vi "Read Points.vi"(8 "error in (no error)":errorcluster, 11 "Locus Recorder in":refnum<class "Locus Recorder.lvclass">) -> (0 "error out":errorcluster, 2 "Points":dbl[][](array[numeric]), 3 "Locus Recorder out":refnum<class "Locus Recorder.lvclass">)   [LabVIEW 2014, in "Locus Recorder.lvclass"]
uses:
  Locus Recorder.lvclass
  Locus Recorder.lvclass/Locus Recorder.ctl
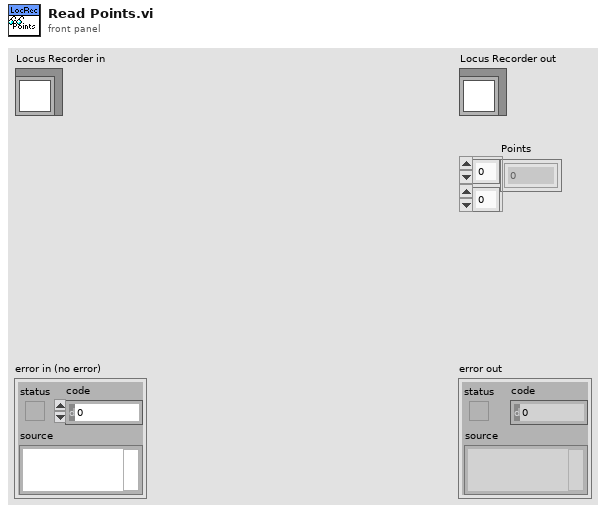
[diagram p1: front panel]
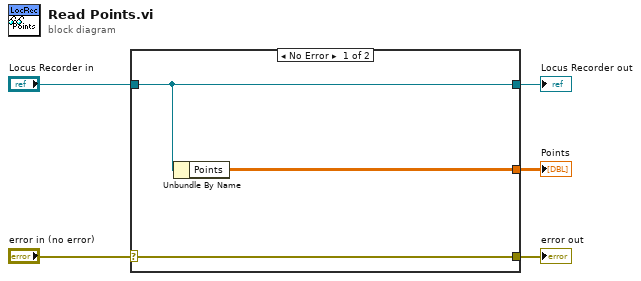
[diagram p0: block diagram]
diagram:
  n1 = case shown="No Error" "error in (no error)" {
    selector: "error in (no error)" -> [w8 w9]
    tunnel: [w8 w9] -> w4
    tunnel: [w7 w10] -> w2
    tunnel: "Locus Recorder in" -> [w7 w10]
    tunnel: [w6 _] -> w1
    frame No Error {
      n2 = Unbundle By Name(w7) -> ("Points"=w6:dbl[][])
    }
    frame Error {
    }
  }
  "error out" <- w4
  "Locus Recorder out" <- w2
  "Points" <- w1
